vi "Inline - Update Status Channels.vi"(7 "Status Channel":T1, 8 "Error Code":i32, 9 "Time (us)":u32, 11 "RTStateVariables":T2 {"RT Inline Data_Data Description_Channels"."Frame Drescriptors"."RT"."Status Channel Ref" format="%.0x"; "RT Inline Data_Data Description_Channels"."Frame Drescriptors"."RT"."Timestamp Channel Data Reference" format="%.0x"; "RT Inline Data_Data Description_Channels"."Frame Drescriptors"."BC"."Status Channel Refs" format="%.0x"; "RT Inline Data_Data Description_Channels"."Frame Drescriptors"."BC"."Timestamp Channel Data Reference" format="%.0x"; "Inline Status Channels Refs" format="%.0x"}) -> ()   [LabVIEW 2017, in "Ballard MIL-1553 Engine.lvlib"]
doc: "This VI updates some Inline Status Channels."
uses:
  Ballard MIL-1553 Engine.lvlib
  Controls/RT StateVariables.ctl
  <vilib>/NI/NIVS Inline Async API/_VS Inline Async API/VS Inline Async API/VS Inline Async API.lvclass
  Controls/Card Parameters.ctl
  Shared/Controls and Global/Initialization Method.ctl
  <vilib>/NI Veristand/Custom Device API/Data Reference.ctl
  Controls/RT Inline Data_Data Description_Channel.ctl
  Controls/RT Inline Frame Descriptor.ctl
  Controls/RT Inline Frame Descriptor_BC.ctl
  <vilib>/NI Veristand/Custom Device API/Block Data Reference.ctl
  <vilib>/NI Veristand/Custom Device API/Custom Device Item Ref.ctl
  Controls/RT Inline Frame Descriptor_RT.ctl
  Shared/Controls and Global/RT CWD2.ctl
  Shared/Controls and Global/RT CWD1.ctl
  Shared/Controls and Global/RT messageType.ctl
  Controls/Inline_Status_Channels.ctl
  <vilib>/NI Veristand/Custom Device API/Global Data Refs.vi
  <vilib>/NI VeriStand/Custom Device API/Custom Device API.lvlib
  Shared/Ballard 1553 Shared.lvlib
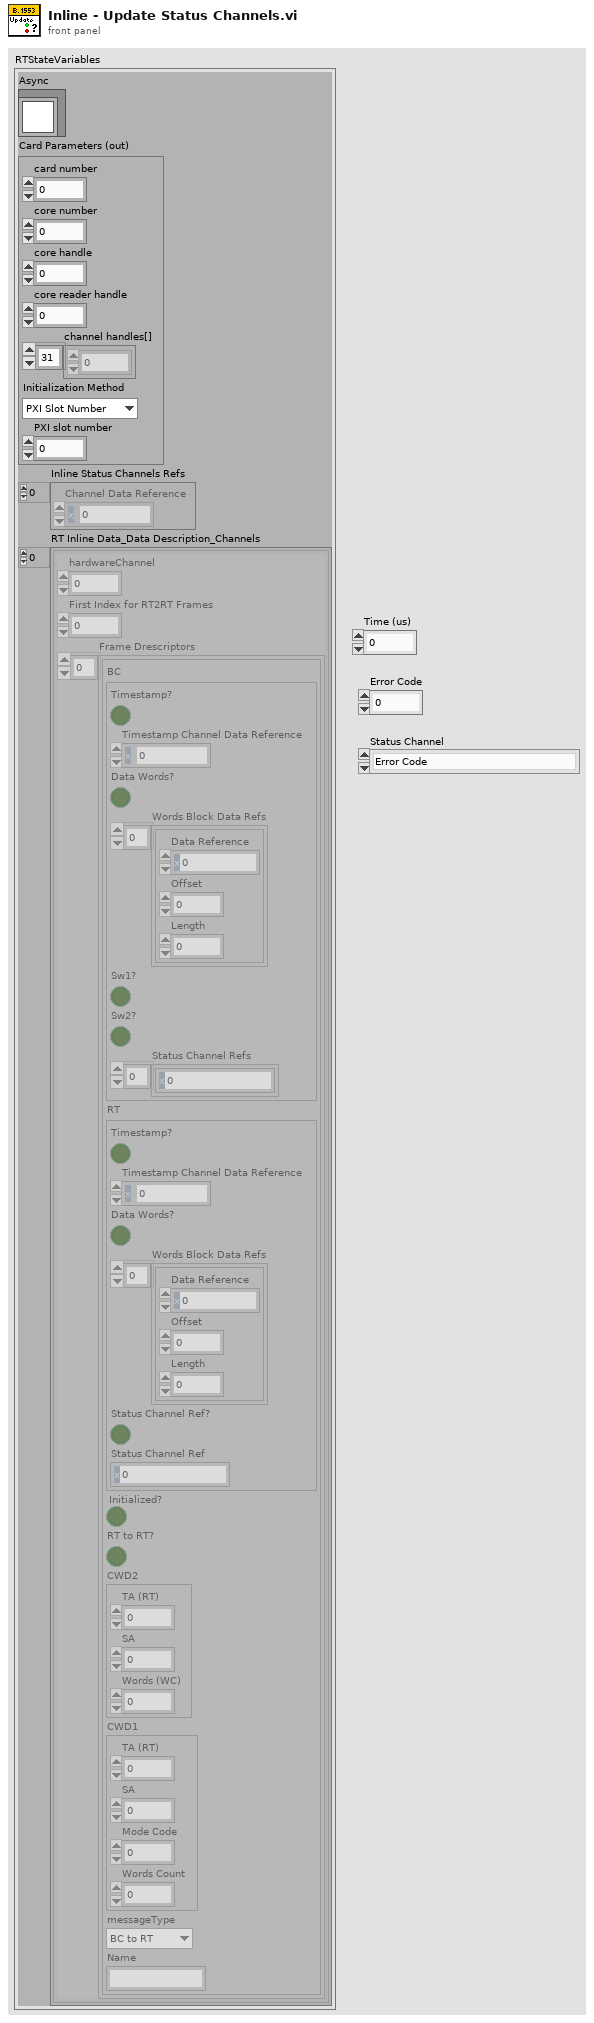
[diagram p1: front panel]
types:
  T1 = typedef "Ballard MIL-1553 Engine.lvlib/Inline_Status_Channels.ctl" = enum16{"Error Code", "Inline Read Time (us)", "Inline Write Time (us)", "Unconfigured Frames Counter", "Monitor - Error Counter", "General Protocol Error Counter", "Wrong Sync Error Counter", "Improper Number of Data Words Error", "Manchester Error Counter", "Parity Error Counter", "Word Error Counter"}
  T2 = typedef "Ballard MIL-1553 Engine.lvlib/RT StateVariables.ctl" = cluster{"Async":refnum<class "VS Inline Async API.lvclass">, "Card Parameters (out)":T3, "Inline Status Channels Refs":T5[], "RT Inline Data_Data Description_Channels":T6[]}
  T3 = typedef "Ballard MIL-1553 Engine.lvlib/Card Parameters.ctl" = cluster{"card number":i32, "core number":i32, "core handle":u64, "core reader handle":u64, "channel handles[]":u64[], "Initialization Method":T4, "PXI slot number":i32}
  T4 = typedef "Ballard 1553 Shared.lvlib/Initialization Method.ctl" = enum16{"PXI Slot Number", "Card Number"}
  T5 = typedef "Custom Device API.lvlib/Data Reference.ctl" = i32
  T6 = typedef "Ballard MIL-1553 Engine.lvlib/RT Inline Data_Data Description_Channel.ctl" = cluster{"hardwareChannel":u16, "First Index for RT2RT Frames":i32, "Frame Drescriptors":T7[]}
  T7 = typedef "Ballard MIL-1553 Engine.lvlib/RT Inline Frame Descriptor.ctl" = cluster{"BC":T8, "RT":T11, "Initialized?":bool, "RT to RT?":bool, "CWD2":T12, "CWD1":T13, "messageType":T14, "Name":string}
  T8 = typedef "Ballard MIL-1553 Engine.lvlib/RT Inline Frame Descriptor_BC.ctl" = cluster{"Timestamp?":bool, "Timestamp Channel Data Reference":T5, "Data Words?":bool, "Words Block Data Refs":T9[], "Sw1?":bool, "Sw2?":bool, "Status Channel Refs":T10[]}
  T9 = typedef "Custom Device API.lvlib/Block Data Reference.ctl" = cluster{"Data Reference":T5, "Offset":u64, "Length":u64}
  T10 = typedef "Custom Device API.lvlib/Custom Device Item Ref.ctl" = u64
  T11 = typedef "Ballard MIL-1553 Engine.lvlib/RT Inline Frame Descriptor_RT.ctl" = cluster{"Timestamp?":bool, "Timestamp Channel Data Reference":T5, "Data Words?":bool, "Words Block Data Refs":T9[], "Status Channel Ref?":bool, "Status Channel Ref":T10}
  T12 = typedef "Ballard 1553 Shared.lvlib/RT CWD2.ctl" = cluster{"TA (RT)":i8, "SA":i8, "Words (WC)":i8}
  T13 = typedef "Ballard 1553 Shared.lvlib/RT CWD1.ctl" = cluster{"TA (RT)":i8, "SA":i8, "Mode Code":i8, "Words Count":i8}
  T14 = typedef "Ballard 1553 Shared.lvlib/RT messageType.ctl" = enum16{"BC to RT", "RT to BC", "RT to RT", "MC (Rx)", "MC (Tx)"}
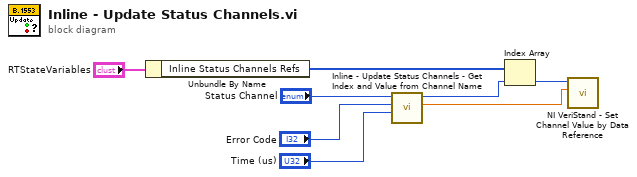
[diagram p0: block diagram]
diagram:
  n1 = Unbundle By Name("RTStateVariables") -> ("Inline Status Channels Refs"=w7:T5[])
  n2 = call "Inline - Update Status Channels - Get Index and Value from Channel Name.vi"("Time (us)/Error Counter Value"="Time (us)", "Error Code"="Error Code", "Status Channel"="Status Channel") -> ("Value"=w2:dbl, "index"=w6:i32)  [unwired: 7 in]
  n3 = Index Array(array=w7, index=w6) -> (element=w5:T5)
  n4 = call <vilib>:"NI VeriStand - Set Channel Value by Data Reference.vi"("Value"=w2, "Data Reference in"=w5) -> ()  [unwired: 9 in, 1 out]
